vi "WinstonAuthAndChipsContent.vi"() -> ()   [LabVIEW 2019]
uses:
  <vilib>/httpClient/POSTBuffer.vi
  <vilib>/httpClient/LabVIEWHTTPClient.lvlib
panel:
  out "jwtToken":string="eyJhbGciOiJIUzI1NiIsInR5cCI6IkpXVCJ9.eyJkYXRhIjp7ImNsaWVudFNlcmlhbCI6ImRldmVsb3BlciIsImxpY2Vuc2VWYWxpZFVudGlsIjoiMTg5NzkxODUyNjAwMCJ9LCJpYXQiOjE1ODIzMDAyMjksImV4cCI6MTU4MjM4NjYyOX0.iY-YLVVzkOAtTILYIx_1T5l_p0eZNRgwxAISscrqsL8"
  out "body":string
  out "headers":string
  in  "IC url":string
  out "error out":errorcluster
  in  "clientSerial":string="developer"
  in  "licenseHash":string
  in  "url":string="https://gikr1vhulg.execute-api.eu-west-1.amazonaws.com/playground/v1/auth/client"
  in  "API key":string
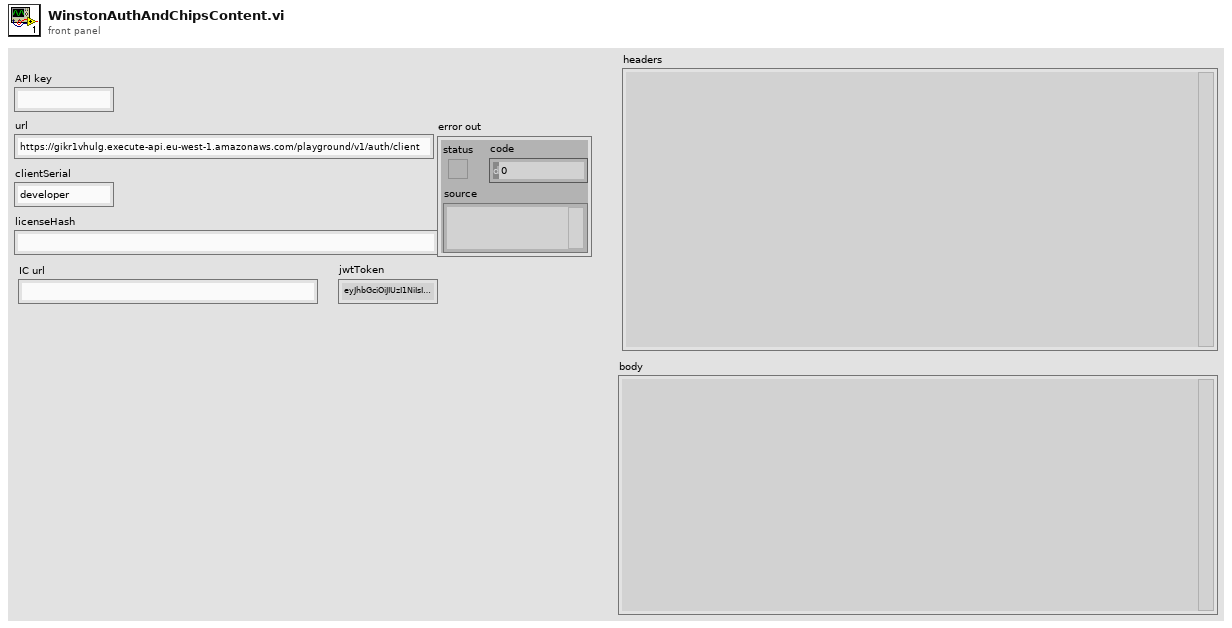
[diagram p1: front panel]
types:
  T1 = cluster{"clientSerial":string, "licenseHash":string}
  T2 = typedef "LabVIEWHTTPClient.lvlib/ClientHandle.ctl" = refnum<k1>
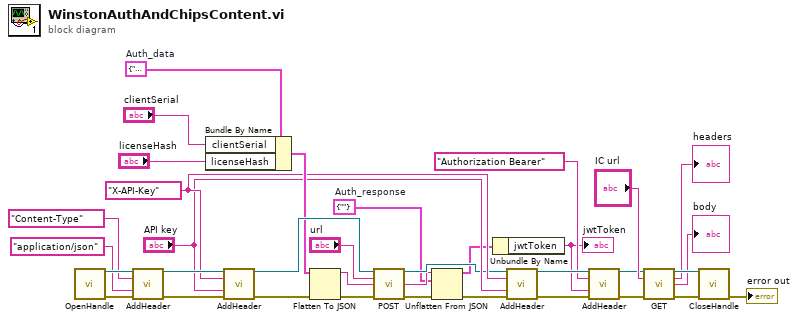
[diagram p0: block diagram]
diagram:
  w4 = cluster{"jwtToken":string} {"jwtToken"=""}  # Auth_response
  w28 = T1 {"clientSerial"="", "licenseHash"=""}  # Auth_data
  w14 = "X-API-Key" ("header")
  n1 = call <vilib>:"OpenHandle.vi"() -> ("client handle out"=w35:T2, "error out"=w34:errorcluster)  [unwired: 14 in]
  n2 = call <vilib>:"AddHeader.vi"("client handle"=w35, "header"="Content-Type", "value"="application/json", "error in (no error)"=w34) -> ("client handle out"=w31:T2, "error out"=w30:errorcluster)  [unwired: 10 in]
  n3 = Bundle By Name(cluster=w28, "clientSerial"="clientSerial", "licenseHash"="licenseHash") -> (w20:T1)
  n4 = call <vilib>:"AddHeader.vi"("client handle"=w31, "header"=w14, "value"="API key", "error in (no error)"=w30) -> ("client handle out"=w24:T2, "error out"=w26:errorcluster)  [unwired: 10 in]
  n5 = Flatten To JSON(anything=w20, error in (no error)=w26) -> (JSON string=w27:string, 11:w25:errorcluster)  [unwired: 1 in]
  n6 = call-poly <vilib>:"POST.vi"("client handle"=w24, "url"="url", "buffer"=w27, "error in (no error)"=w25) -> ("client handle out"=w12:T2, "body"=w11:string, "error out"=w23:errorcluster)  [unwired: 8 in, 1 out]
  n7 = Unflatten From JSON(JSON string=w11, type and defaults=w4, error in (no error)=w23) -> (value=w3:cluster{"jwtToken":string}, error out=w2:errorcluster)  [unwired: 4 in]
  n8 = Unbundle By Name(w3) -> ("jwtToken"=w1:string)
  "jwtToken" <- w1
  n9 = call <vilib>:"AddHeader.vi"("client handle"=w12, "header"=w14, "value"="API key", "error in (no error)"=w2) -> ("client handle out"=w10:T2, "error out"=w5:errorcluster)  [unwired: 10 in]
  n10 = call <vilib>:"AddHeader.vi"("client handle"=w10, "header"="Authorization Bearer", "value"=w1, "error in (no error)"=w5) -> ("client handle out"=w9:T2, "error out"=w6:errorcluster)  [unwired: 10 in]
  n11 = call <vilib>:"GET.vi"("client handle"=w9, "url"="IC url", "error in (no error)"=w6) -> ("client handle out"=w18:T2, "headers"=→"headers":string, "body"=→"body":string, "error out"=w7:errorcluster)  [unwired: 9 in]
  n12 = call <vilib>:"CloseHandle.vi"("client handle"=w18, "error in (no error)"=w7) -> ("error out"=→"error out":errorcluster)  [unwired: 13 in]
